vi "Draw ID COB-ID and OD Idx Columns.vi"(7 "PDO Slot Index":i32, 8 "error in":errorcluster, 9 "PDO Slot in":refnum<class "PDO Slot.lvclass">, 10 "Row":i32, 11 "PDO Grid in":refnum<class "PDO Grid.lvclass">) -> (0 "error out":errorcluster, 3 "PDO Grid out":refnum<class "PDO Grid.lvclass">)   [LabVIEW 2019, in "PDO Grid.lvlib" / "PDO Grid.lvclass"]
uses:
  PDO Grid.lvclass
  D:/git/Sourcegrid-LabVIEW/source/Grid/SourceGrid.lvclass
  PDO Slot/PDO Slot.lvclass
  Sourcegrid-LabVIEW/source/Cells/Cell/Cell.lvclass
  Sourcegrid-LabVIEW/source/Views/Cell View Alternating Back Color/Cell View Alternating Back Color.lvclass
  D:/git/Sourcegrid-LabVIEW/source/Views/Cell View/Cell View.lvclass
  Sourcegrid-LabVIEW/source/System.Drawing.Color.ctl
  Sourcegrid-LabVIEW/source/SourceGrid.lvlib
  Sourcegrid-LabVIEW/source/Grid/SourceGrid.lvclass
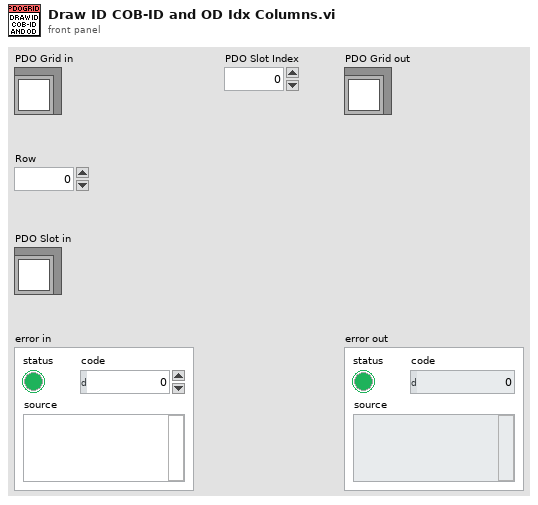
[diagram p1: front panel]
types:
  T1 = typedef "SourceGrid.lvlib/System.Drawing.Color.ctl" = enum16{"AliceBlue", "AntiqueWhite", "Aqua", "Aquamarine", "Azure", "Beige", "Bisque", "Black", "BlanchedAlmond", "Blue", "BlueViolet", "Brown", "BurlyWood", "CadetBlue", "Chartreuse", "Chocolate", "Coral", "CornflowerBlue", "Cornsilk", "Crimson", "Cyan", "DarkBlue", "DarkCyan", "DarkGoldenrod", "DarkGray", "DarkGreen", "DarkKhaki", "DarkMagenta", "DarkOliveGreen", "DarkOrange", "DarkOrchid", "DarkRed", "DarkSalmon", "DarkSeaGreen", "DarkSlateBlue", "DarkSlateGray", "DarkTurquoise", "DarkViolet", "DeepPink", "DeepSkyBlue", "DimGray", "DodgerBlue", "Firebrick", "FloralWhite", "ForestGreen", "Fuchsia", "Gainsboro", "GhostWhite", "Gold", "Goldenrod", "Gray", "Green", "GreenYellow", "Honeydew", "HotPink", "IndianRed", "Indigo", "Ivory", "Khaki", "Lavender", "LavenderBlush", "LawnGreen", "LemonChiffon", "LightBlue", "LightCoral", "LightCyan", "LightGoldenrodYellow", "LightGray", "LightGreen", "LightPink", "LightSalmon", "LightSeaGreen", "LightSkyBlue", "LightSlateGray", "LightSteelBlue", "LightYellow", "Lime", "LimeGreen", "Linen", "Magenta", "Maroon", "MediumAquamarine", "MediumBlue", "MediumOrchid", "MediumPurple", "MediumSeaGreen", "MediumSlateBlue", "MediumSpringGreen", "MediumTurquoise", "MediumVioletRed", "MidnightBlue", "MintCream", "MistyRose", "Moccasin", "NavajoWhite", "Navy", "OldLace", "Olive", "OliveDrab", "Orange", "OrangeRed", "Orchid", "PaleGoldenrod", "PaleGreen", "PaleTurquoise", "PaleVioletRed", "PapayaWhip", "PeachPuff", "Peru", "Pink", "Plum", "PowderBlue", "Purple", "Red", "RosyBrown", "RoyalBlue", "SaddleBrown", "Salmon", "SandyBrown", "SeaGreen", "SeaShell", "Sienna", "Silver", "SkyBlue", "SlateBlue", "SlateGray", "Snow", "SpringGreen", "SteelBlue", "Tan", "Teal", "Thistle", "Tomato", "Transparent", "Turquoise", "Violet", "Wheat", "White", "WhiteSmoke", "Yellow"}
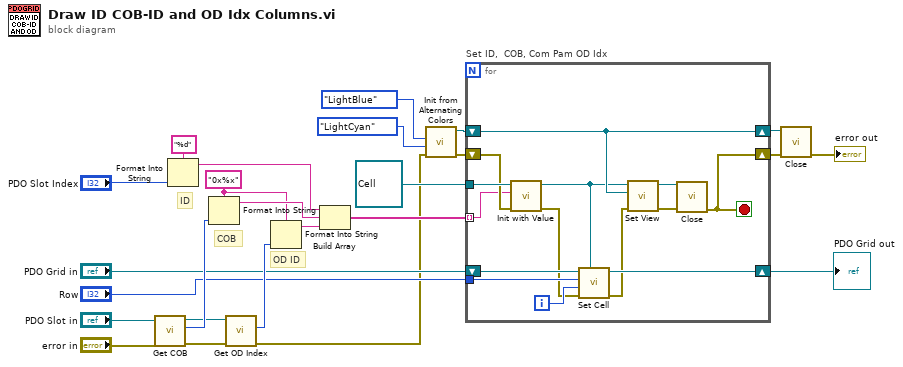
[diagram p0: block diagram]
diagram:
  w16 = "0x%x" ("format string")
  # "OD ID"
  # "COB"
  # "ID"
  n1 = call "Get COB.vi"("error in"="error in", "PDO Slot in"="PDO Slot in") -> ("error out"=w17:errorcluster, "COB-ID"=w15:u32, "PDO Slot out"=w14:refnum<class "PDO Slot.lvclass">)  [unwired: 7 in]
  n2 = Format Into String(format string="%d", "PDO Slot Index") -> (resulting string=w21:string)  [unwired: 2 in, 1 out]
  n3 = Format Into String(format string=w16, w15) -> (resulting string=w20:string)  [unwired: 2 in, 1 out]
  n4 = call "Get OD Index.vi"("error in"=w17, "PDO Slot in"=w14) -> ("error out"=w4:errorcluster, "OD Index"=w18:u16)  [unwired: 7 in, 1 out]
  n5 = Format Into String(format string=w16, w18) -> (resulting string=w19:string)  [unwired: 2 in, 1 out]
  n6 = Build Array(w21, w20, w19) -> (w22:string[])
  n7 = call "Init from Alternating Colors.vi"("error in"=w4, "Color Not Equal"=System.Drawing.Color."LightCyan" ("Color"), "Color Equal"=System.Drawing.Color."LightBlue" ("Color")) -> ("error out"=w3:errorcluster, "Cell View Alternating Back Color out"=w5:refnum<class "Cell View Alternating Back Color.lvclass">)  [unwired: 7 in]
  n8 = for "Set ID,  COB, Com Pam OD Idx" {
    tunnel: "Row" -> [w34]
    tunnel: refnum<class "Cell.lvclass"> refnum ("SourceGrid.lvlib:Cell.lvclass") -> [w37]
    tunnel: w22 -> [w31] mode=indexing
    shift-right: [w36] -> w8
    shift-left: w3 -> [w33]
    shift-right: [w38] -> w24
    shift-left: "PDO Grid in" -> [w39]
    shift-right: [w27] -> w1
    shift-left: w5 -> [w27]
    i -> [w35]
    stop <- w36 stop-if-true
    n9 = call-dynamic "Init with Value.vi"("error in"=w33, "Value"=w31, "Cell in"=w37) -> ("error out"=w32:errorcluster, "Cell out"=w26:refnum<class "Cell.lvclass">)  [unwired: 7 in]
    n10 = call "Set Cell.vi"("Cell"=w26, "error in"=w32, "Column"=w35, "Row"=w34, "Sourcegrid in"=w39) -> ("error out"=w30:errorcluster, "Sourcegrid out"=w38:refnum<class "PDO Grid.lvclass">)  [unwired: 5 in]
    n11 = call-dynamic "Set View.vi"("error in"=w30, "CellView"=w27, "Cell in"=w26) -> ("error out"=w29:errorcluster, "Cell out"=w28:refnum<class "Cell.lvclass">)  [unwired: 7 in]
    n12 = call-dynamic "Close.vi"("error in"=w29, "Cell in"=w28) -> ("error out"=w36:errorcluster)  [unwired: 8 in, 1 out]
  }
  "PDO Grid out" <- w24
  n13 = call-dynamic "Close.vi"("error in"=w8, "Cell View Alternating Back Color in"=w1) -> ("error out"=→"error out":errorcluster)  [unwired: 8 in, 1 out]
